vi "File Page - Get Advanced Settings.vi"(7 "File Ctl Refs":T1, 8 "error in (no error)":errorcluster, 11 "Item Ref in":T11 format="%.0x") -> (0 "error out":errorcluster, 3 "Item Ref out":T11 format="%.0x")   [LabVIEW 2012, in "Waveform Data Logger System Explorer.lvlib"]
uses:
  Waveform Data Logger System Explorer.lvlib
  <vilib>/NI Veristand/Custom Device API/Custom Device Item Ref.ctl
  Types/File Ctl Refs.ctl
  Types/File - Spec Ctl Refs.ctl
  Types/File - Wfm Ctl Refs.ctl
  Types/File - Settings Ctl Refs.ctl
  Shared/Classes/Log File Specifications/Log File Specification/File Conflict Operation.ctl
  Types/File - Start Trig Ctl Refs.ctl
  Shared/Types/Start Trigger.ctl
  Shared/Types/Default Trigger.ctl
  Shared/Types/Digital Trigger.ctl
  Shared/Types/Analog Trigger.ctl
  Shared/Types/In Range Trigger.ctl
  Shared/Types/Value Change Trigger.ctl
  Shared/Types/Boolean Trigger.ctl
  Types/Single Node Browser Data.ctl
  <vilib>/NI Veristand/UI Controls/Single Node Browser/Single Node Browser Ref.ctl
  NationalInstruments.VeriStand.SystemStorageUI
  <vilib>/NI Veristand/UI Controls/Single Node Browser/Callback Type.ctl
  <vilib>/NI Veristand/UI Controls/Single Node Browser/Net Event Data.ctl
  <vilib>/NI Veristand/UI Controls/Single Node Browser/Net Event.ctl
  Types/File - Stop Trig Ctl Refs.ctl
  Shared/Types/Stop Trigger.ctl
  Types/File - Advanced Ctl Refs.ctl
  Types/Log Timestamps.ctl
  Shared/Globals/Property Strings.vi
  <vilib>/NI Veristand/Custom Device API/Get Item Property (Double).vi
  <vilib>/NI Veristand/Custom Device API/Get Item Property (Boolean).vi
  <vilib>/NI Veristand/Custom Device API/Get Item Property (U32).vi
  <vilib>/NI Veristand/Custom Device API/Custom Device API.lvlib
  Shared/Waveform Data Logger Shared.lvlib
  Shared/Classes/Log File Specifications/Log File Specification/Log File Specification.lvclass
  <vilib>/NI Veristand/UI Controls/Single Node Browser/NI_VS UI Single Node Browser.lvlib
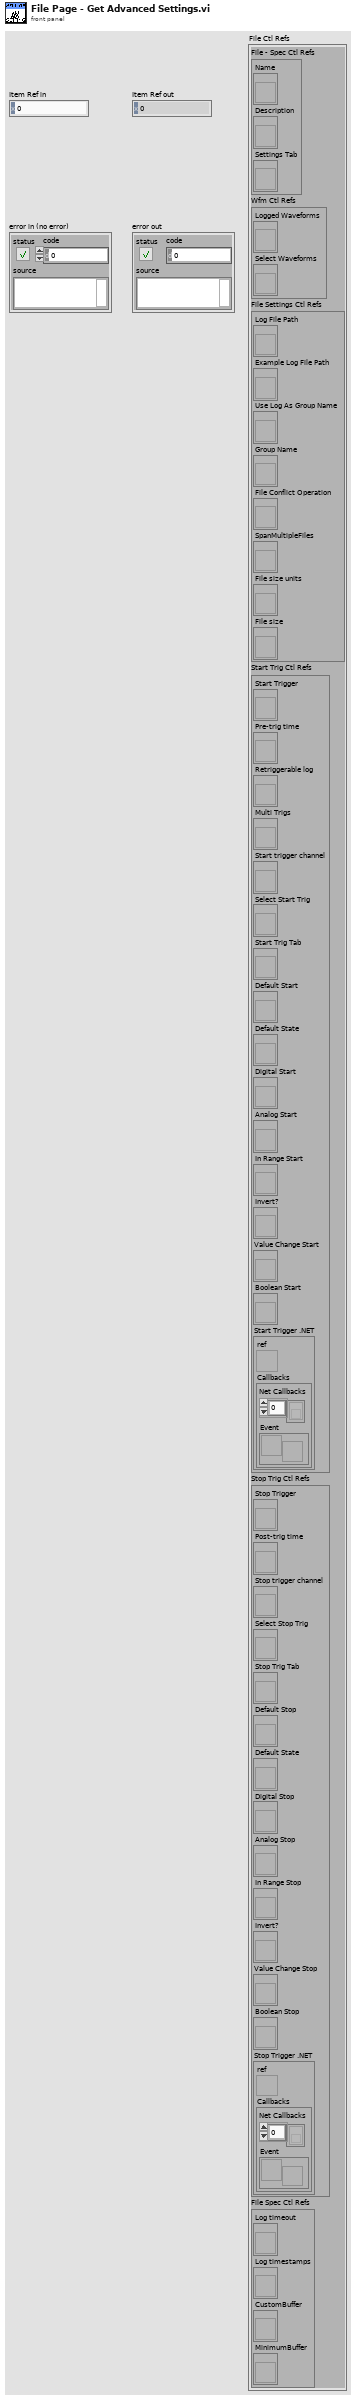
[diagram p1: front panel]
types:
  T1 = typedef "Waveform Data Logger System Explorer.lvlib/File Ctl Refs.ctl" = cluster{"File Spec Ctl Refs":T2, "Wfm Ctl Refs":T3, "File Settings Ctl Refs":T4, "Start Trig Ctl Refs":T5, "Stop Trig Ctl Refs":T9, "File Spec Ctl Refs":T10}
  T2 = typedef "Waveform Data Logger System Explorer.lvlib/File - Spec Ctl Refs.ctl" = cluster{"Name":refnum<vi>, "Description":refnum<vi>, "Settings Tab":refnum<vi>}
  T3 = typedef "Waveform Data Logger System Explorer.lvlib/File - Wfm Ctl Refs.ctl" = cluster{"Logged Waveforms":refnum<vi>, "Select Waveforms":refnum<vi>}
  T4 = typedef "Waveform Data Logger System Explorer.lvlib/File - Settings Ctl Refs.ctl" = cluster{"Log File Path":refnum<vi>, "Example Log File Path":refnum<vi>, "Use Log As Group Name":refnum<vi>, "Group Name":refnum<vi>, "File Conflict Operation":refnum<vi>, "SpanMultipleFiles":refnum<vi>, "File size units":refnum<vi>, "File size":refnum<vi>}
  T5 = typedef "Waveform Data Logger System Explorer.lvlib/File - Start Trig Ctl Refs.ctl" = cluster{"Start Trigger":refnum<vi>, "Pre-trig time":refnum<vi>, "Retriggerable log":refnum<vi>, "Multi Trigs":refnum<vi>, "Start trigger channel":refnum<vi>, "Select Start Trig":refnum<vi>, "Start Trig Tab":refnum<vi>, "Default Start":refnum<vi>, "Default State":refnum<vi>, "Digital Start":refnum<vi>, "Analog Start":refnum<vi>, "In Range Start":refnum<vi>, "Invert?":refnum<vi>, "Value Change Start":refnum<vi>, "Boolean Start":refnum<vi>, "Start Trigger .NET":T6}
  T6 = typedef "Waveform Data Logger System Explorer.lvlib/Single Node Browser Data.ctl" = cluster{"ref":T7, "Callbacks":T8}
  T7 = typedef "NI_VS UI Single Node Browser.lvlib/Single Node Browser Ref.ctl" = refnum<k24>
  T8 = typedef "NI_VS UI Single Node Browser.lvlib/Callback Type.ctl" = cluster{"Net Callbacks":refnum<k27>[], "Event":refnum<user-event>}
  T9 = typedef "Waveform Data Logger System Explorer.lvlib/File - Stop Trig Ctl Refs.ctl" = cluster{"Stop Trigger":refnum<vi>, "Post-trig time":refnum<vi>, "Stop trigger channel":refnum<vi>, "Select Stop Trig":refnum<vi>, "Stop Trig Tab":refnum<vi>, "Default Stop":refnum<vi>, "Default State":refnum<vi>, "Digital Stop":refnum<vi>, "Analog Stop":refnum<vi>, "In Range Stop":refnum<vi>, "Invert?":refnum<vi>, "Value Change Stop":refnum<vi>, "Boolean Stop":refnum<vi>, "Stop Trigger .NET":T6}
  T10 = typedef "Waveform Data Logger System Explorer.lvlib/File - Advanced Ctl Refs.ctl" = cluster{"Log timeout":refnum<vi>, "Log timestamps":refnum<vi>, "CustomBuffer":refnum<vi>, "MinimumBuffer":refnum<vi>}
  T11 = typedef "Custom Device API.lvlib/Custom Device Item Ref.ctl" = u64
  T12 = enum8{"Enabled", "Disabled", "Disabled and Grayed Out"}
  T13 = typedef "Waveform Data Logger System Explorer.lvlib/Log Timestamps.ctl" = enum16{"Use waveform timestamps", "Timestamp based on when data is received by the logger"}
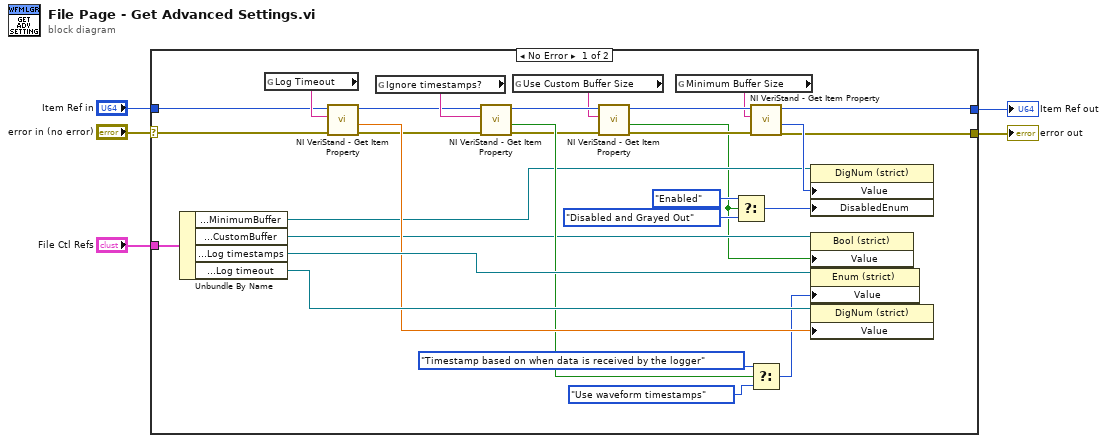
[diagram p0: block diagram]
diagram:
  n1 = case shown="No Error" "error in (no error)" {
    selector: "error in (no error)" -> [w29 w35]
    tunnel: [w11 w36] -> w5
    tunnel: [w10 w35] -> w4
    tunnel: "Item Ref in" -> [w30 w36]
    tunnel: "File Ctl Refs" -> [w34 _]
    frame No Error {
      n2 = Unbundle By Name(w34) -> ("File Spec Ctl Refs.MinimumBuffer"=w12:refnum<vi>, "File Spec Ctl Refs.CustomBuffer"=w17:refnum<vi>, "File Spec Ctl Refs.Log timestamps"=w32:refnum<vi>, "File Spec Ctl Refs.Log timeout"=w33:refnum<vi>)
      n3 = global read "Property Strings.vi" "Log Timeout"() -> (w31:string)
      n4 = call-poly <vilib>:"NI VeriStand - Get Item Property.vi"("error in (no error)"=w29, "Property Name"=w31, "Item Ref in"=w30) -> ("error out"=w22:errorcluster, "Value"=w28:dbl, "Item Ref out"=w23:T11)  [unwired: 1 in, 5 out]
      n5 = global read "Property Strings.vi" "Ignore timestamps?"() -> (w24:string)
      n6 = call-poly <vilib>:"NI VeriStand - Get Item Property.vi"("error in (no error)"=w22, "Property Name"=w24, "Item Ref in"=w23) -> ("error out"=w19:errorcluster, "Value"=w21:bool, "Item Ref out"=w20:T11)  [unwired: 1 in, 5 out]
      n7 = global read "Property Strings.vi" "Use Custom Buffer Size"() -> (w18:string)
      n8 = call-poly <vilib>:"NI VeriStand - Get Item Property.vi"("error in (no error)"=w19, "Property Name"=w18, "Item Ref in"=w20) -> ("error out"=w16:errorcluster, "Value"=w6:bool, "Item Ref out"=w15:T11)  [unwired: 1 in, 5 out]
      n9 = global read "Property Strings.vi" "Minimum Buffer Size"() -> (w14:string)
      n10 = Select(t=T12."Enabled" ("Disabled"), s=w6, f=T12."Disabled and Grayed Out" ("Disabled")) -> (s? t:f=w7:T12)
      n11 = call-poly <vilib>:"NI VeriStand - Get Item Property.vi"("error in (no error)"=w16, "Property Name"=w14, "Item Ref in"=w15) -> ("error out"=w10:errorcluster, "Value"=w13:u32, "Item Ref out"=w11:T11)  [unwired: 1 in, 5 out]
      n12 = Select(t=Log_Timestamps."Timestamp based on when data is received by the logger" ("Log timestamps"), s=w21, f=Log_Timestamps."Use waveform timestamps" ("Log timestamps")) -> (s? t:f=w25:T13)
      n13 = property class="DigNum (strict)"(reference=w12, "Value"=w13, "DisabledEnum"=w7) -> ()  [unwired: 1 in, 2 out]
      n14 = property class="Bool (strict)"(reference=w17, "Value"=w6) -> ()  [unwired: 1 in, 2 out]
      n15 = property class="Enum (strict)"(reference=w32, "Value"=w25) -> ()  [unwired: 1 in, 2 out]
      n16 = property class="DigNum (strict)"(reference=w33, "Value"=w28) -> ()  [unwired: 1 in, 2 out]
    }
    frame Error {
    }
  }
  "error out" <- w4
  "Item Ref out" <- w5
